vi "voltagePrecentage.vi"(11 "Numeric":sgl) -> (1 "Boolean 2":bool, 2 "Boolean 3":bool, 3 "Boolean 4":bool, 4 "Boolean":bool)   [LabVIEW 2015]
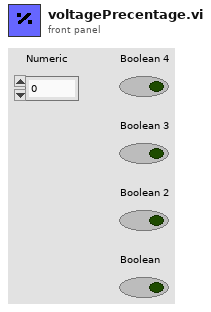
[diagram p1: front panel]
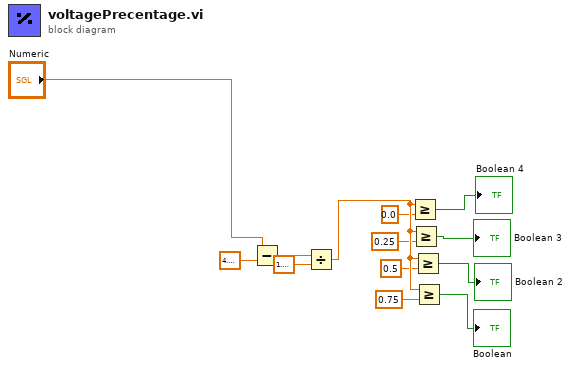
[diagram p0: block diagram]
diagram:
  n1 = Subtract(x="Numeric", y=sgl 4.8) -> (x-y=w3:sgl)
  n2 = Divide(x=w3, y=sgl 1.4) -> (x/y=w9:sgl)
  n3 = Greater Or Equal?(x=w9, y=0.0) -> (x >= y?=→"Boolean 4":bool)
  n4 = Greater Or Equal?(x=w9, y=0.25) -> (x >= y?=→"Boolean 3":bool)
  n5 = Greater Or Equal?(x=w9, y=0.5) -> (x >= y?=→"Boolean 2":bool)
  n6 = Greater Or Equal?(x=w9, y=0.75) -> (x >= y?=→"Boolean":bool)
